vi "VDH-generateCalibrationSOLT.vi"(8 "error in (no error)":errorcluster, 11 "VDH-VNA_data_handler in":refnum<class "VDH-VNA_data_handler.lvclass">) -> (0 "error out":errorcluster, 3 "VDH-VNA_data_handler out":refnum<class "VDH-VNA_data_handler.lvclass">)   [LabVIEW 2020, in "VDH-VNA_data_handler.lvlib" / "VDH-VNA_data_handler.lvclass"]
uses:
  VDH-VNA_data_handler.lvclass
  VDH-VNA_data_handler.lvclass/VDH-VNA_data_handler.ctl
  VDH-Calibration_prosess.ctl
  VDH-Calibration_enum.ctl
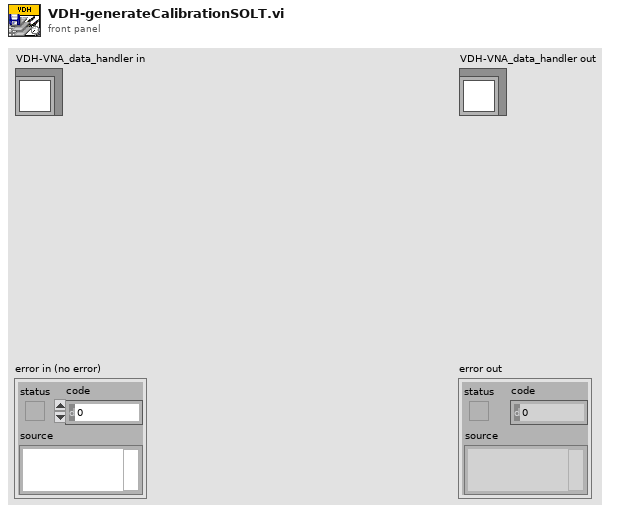
[diagram p1: front panel]
types:
  T1 = typedef "VDH-VNA_data_handler.lvlib/VDH-VNA_data_handler.lvclass/VDH-Calibration_prosess.ctl" = cluster{"Progress":bool, "current":T2, "samples to get":u8}
  T2 = typedef "VDH-VNA_data_handler.lvlib/VDH-VNA_data_handler.lvclass/VDH-Calibration_enum.ctl" = enum16{"Non", "Short", "Open", "Load", "Through", "Permativity"}
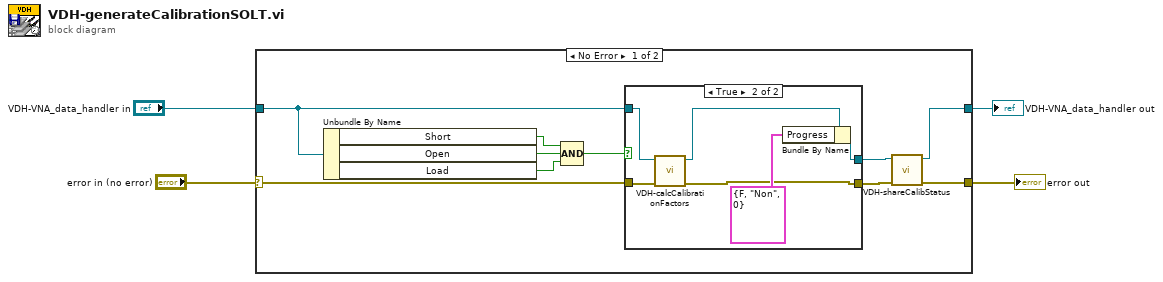
[diagram p0: block diagram]
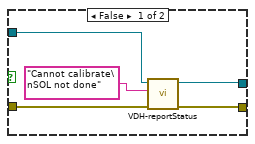
[diagram p2: hidden frame]
diagram:
  n1 = case shown="No Error" "error in (no error)" {
    selector: "error in (no error)" -> [w9 w27]
    tunnel: [w7 w27] -> w3
    tunnel: [w5 w26] -> w1
    tunnel: "VDH-VNA_data_handler in" -> [w11 w26]
    frame No Error {
      n2 = Unbundle By Name(w11) -> ("Short"=w14:bool, "Open"=w13:bool, "Load"=w12:bool)
      n3 = Compound Arithmetic op=AND(w14, w13, w12) -> (w10:bool)
      n4 = case shown="True" w10 {
        tunnel: w11 -> [w17 w20]
        tunnel: [w16 w23] -> w6
        tunnel: w9 -> [w18 w25]
        tunnel: [w19 w22] -> w8
        frame False {
          n5 = call "VDH-reportStatus.vi"("error in (no error)"=w18, "message"="Cannot calibrate\nSOL not done", "VDH-VNA_data_handler in"=w17) -> ("error out"=w19:errorcluster, "VDH-VNA_data_handler out"=w16:refnum<class "VDH-VNA_data_handler.lvclass">)  [unwired: 7 in]
        }
        frame True {
          n6 = call "VDH-calcCalibrationFactors.vi"("error in (no error)"=w25, "VDH-VNA_data_handler in"=w20) -> ("error out"=w22:errorcluster, "VDH-VNA_data_handler out"=w21:refnum<class "VDH-VNA_data_handler.lvclass">)  [unwired: 8 in]
          n7 = Bundle By Name(cluster=w21, "Progress"=T1 {"Progress"=FALSE, "current"=enum."Non", "samples to get"=0} ("Calibration Status.Progress")) -> (w23:refnum<class "VDH-VNA_data_handler.lvclass">)
        }
      }
      n8 = call "VDH-shareCalibStatus.vi"("error in (no error)"=w8, "VDH-VNA_data_handler in"=w6) -> ("error out"=w7:errorcluster, "VDH-VNA_data_handler out"=w5:refnum<class "VDH-VNA_data_handler.lvclass">)  [unwired: 8 in]
    }
    frame Error {
    }
  }
  "error out" <- w3
  "VDH-VNA_data_handler out" <- w1
